vi "AO Reg UI.vi"(8 "error in (no error)":errorcluster, 11 "Node Ptr":T4 format="%.0x") -> (0 "error out":errorcluster)   [LabVIEW 2019, in "Modbus Master System Explorer.lvlib"]
uses:
  Modbus Master System Explorer.lvlib
  <vilib>/NI VeriStand/Custom Device API/Custom Device Item Ref.ctl
  Shared/Controls/Data Model/DataType.ctl
  SubVIs/Radix.ctl
  SubVIs/Direction.ctl
  <vilib>/NI VeriStand/Custom Device API/Custom Device API.lvlib
  Shared/Modbus Master Shared.lvlib
panel:
  in  "Default Value":dbl
  in  "Direction":T1
  in  "Radix":T2
  out "Registers":i32
  in  "Sub-Index (Bool)":u16
  in  "DataType":T3
  in  "Valid?":string
  in  "Address":u16
  in  "Header":cluster{"Section Name":string}={"Section Name"="Holding Register (Analog Out) Settings"}
  in  "Description":string
  in  "Name":string
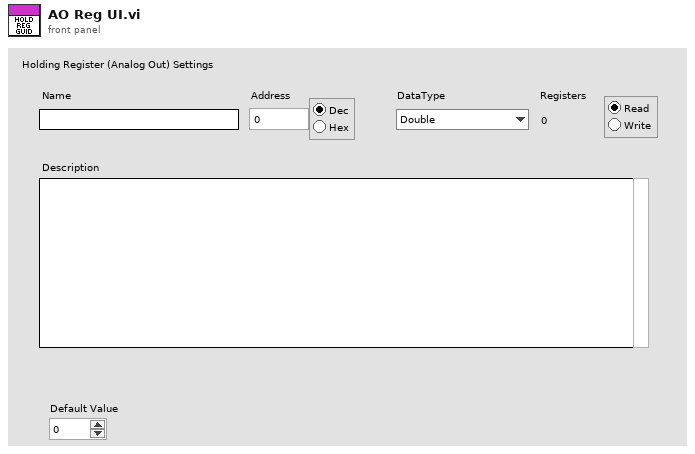
[diagram p1: front panel]
types:
  T1 = typedef "Modbus Master System Explorer.lvlib/Direction.ctl" = enum32{"Radio Selection 1", "Radio Selection 2"}
  T2 = typedef "Modbus Master System Explorer.lvlib/Radix.ctl" = enum32{"Decimal", "Hexidecimal"}
  T3 = typedef "Modbus Master Shared.lvlib/DataType.ctl" = enum16{"Double", "Single", "I64", "I32", "I16", "I8", "U64", "U32", "U16", "U8", "Boolean"}
  T4 = typedef "Custom Device API.lvlib/Custom Device Item Ref.ctl" = u64
  T5 = enum8{"Enabled", "Disabled", "Disabled and Grayed Out"}
  T6 = typedef "Custom Device API.lvlib/Custom Device Commands.ctl" = enum16{"Default", "Item renamed", "Shutdown", "Dynamic button pressed"}
  T7 = typedef "Custom Device API.lvlib/Custom Device Item Info.ctl" = cluster{"Name":string, "Is Channel":bool, "GUID":string, "Is Waveform":bool}
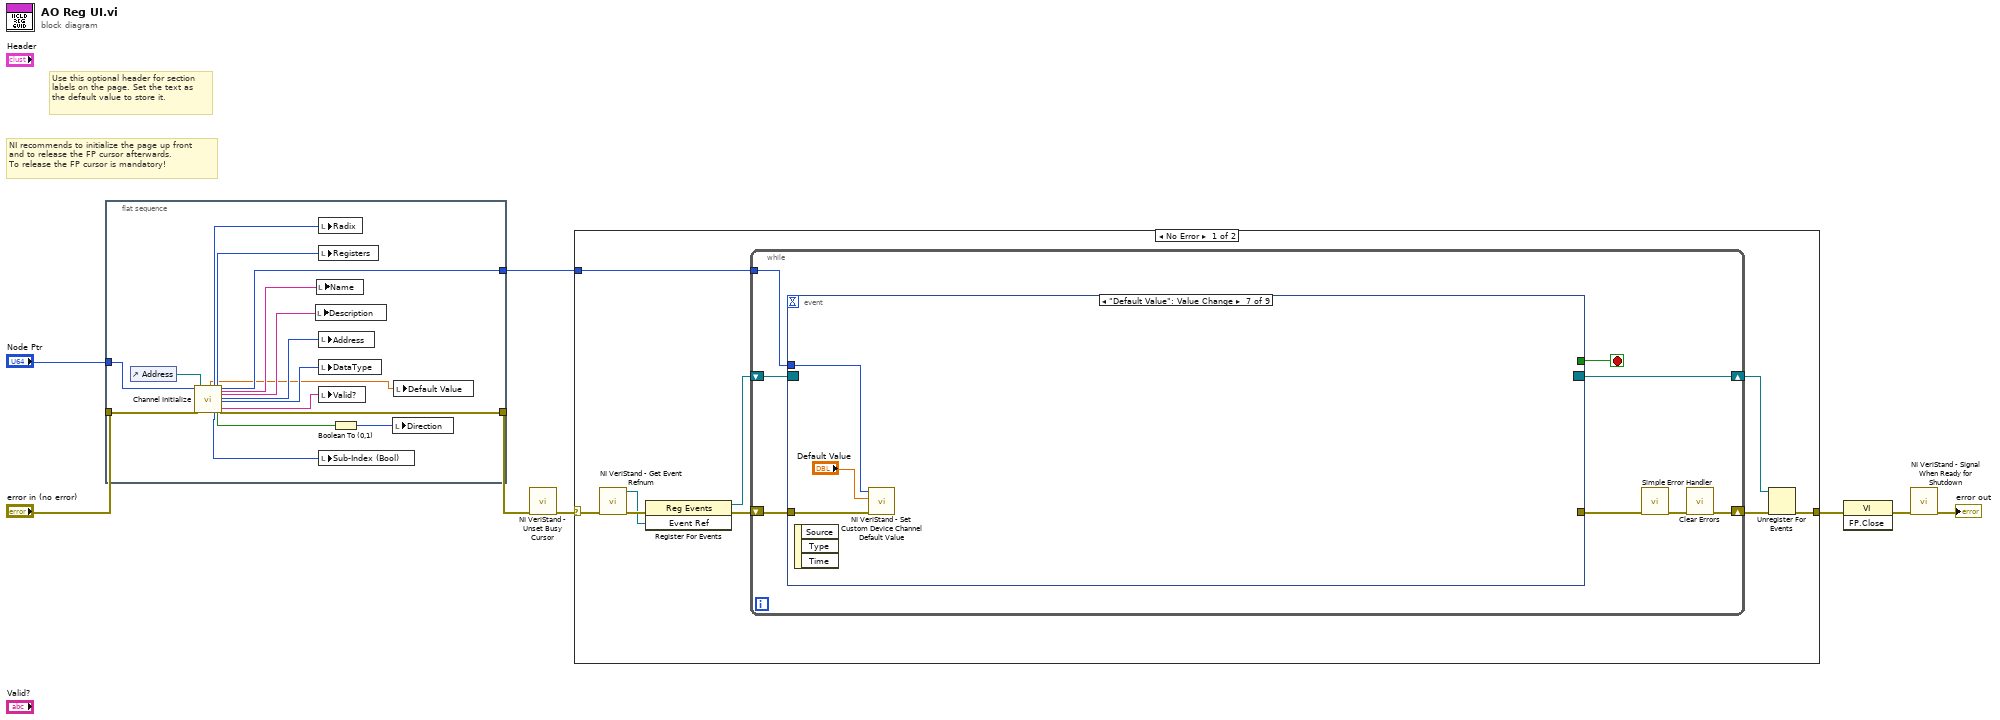
[diagram p0: block diagram]
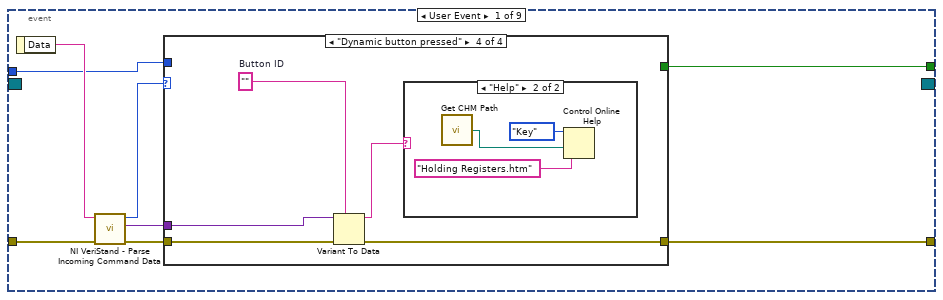
[diagram p2: hidden frame]
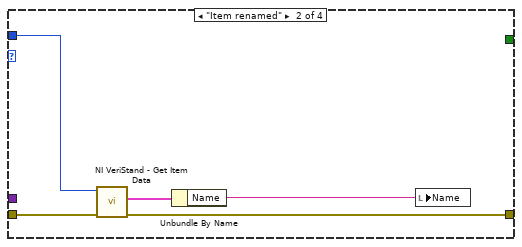
[diagram p4: hidden frame]
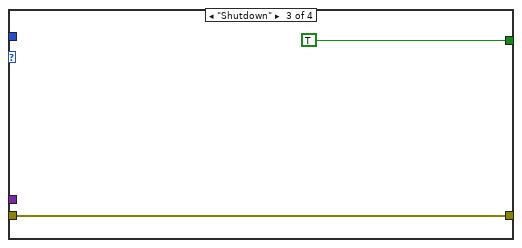
[diagram p5: hidden frame]
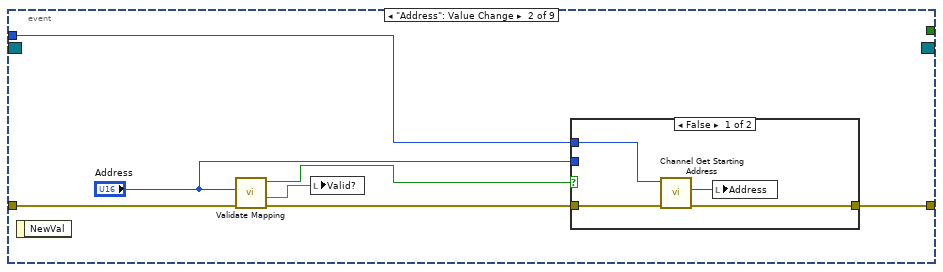
[diagram p7: hidden frame]
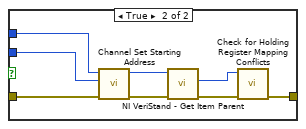
[diagram p8: hidden frame]
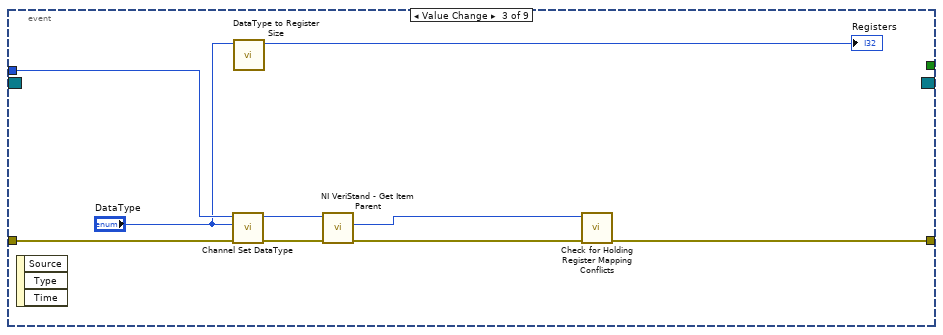
[diagram p9: hidden frame]
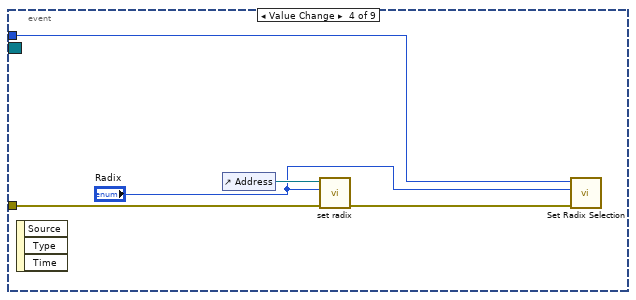
[diagram p10: hidden frame]
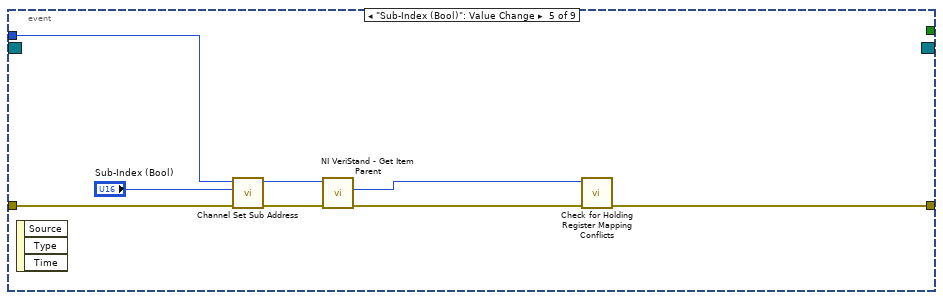
[diagram p11: hidden frame]
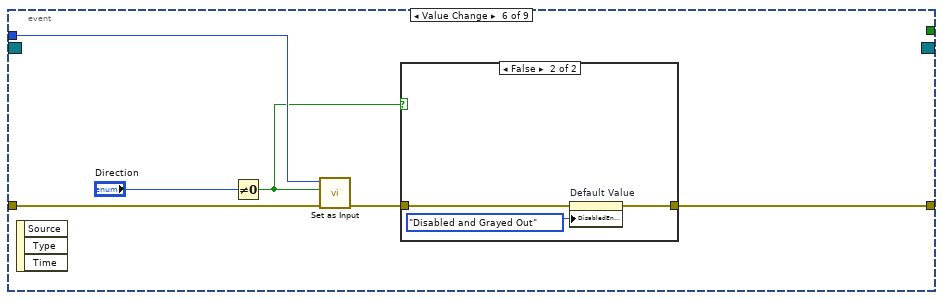
[diagram p12: hidden frame]
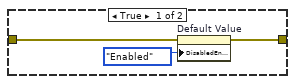
[diagram p13: hidden frame]
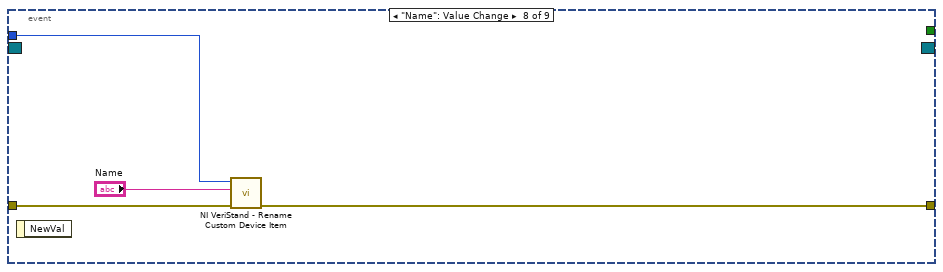
[diagram p14: hidden frame]
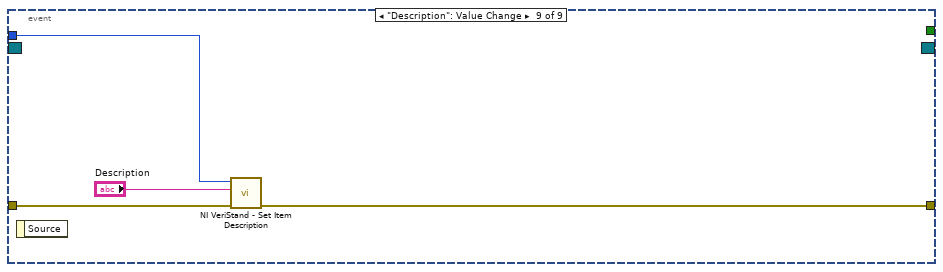
[diagram p15: hidden frame]
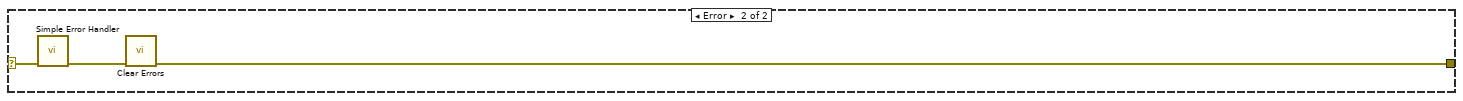
[diagram p16: hidden frame]
diagram:
  # "Use this optional header for section labels on the page. Set the text as the default value to store it."
  # "NI recommends to initialize the page up front\nand to release the FP cursor afterwards.\nTo release the FP cursor is mandatory!"
  n1 = flat-sequence {
    tunnel: "Node Ptr" -> [w13]
    tunnel: "error in (no error)" -> [w12]
    tunnel: [w11] -> w2
    tunnel: [w10] -> w1
    frame #0 {
      n2 = control-ref of="Address"() -> (w17:refnum<vi>)
      n3 = call "Channel Initialize.vi"("Item Ref in"=w13, "error in (no error)"=w12, "Starting Address Ref in"=w17) -> ("Default Value"=w9:dbl, "Radix"=w16:T2, "Sub-Index (Bool)"=w19:u16, "Registers"=w20:i32, "input?"=w14:bool, "Channel Ref out"=w11:T4, "Name"=w23:string, "Description"=w24:string, "Starting Address"=w21:u16, "DataType"=w22:T3, "Status Message"=w18:string, "error out"=w10:errorcluster)  [unwired: 12 in, 1 out]
      n4 = local write "Description"(w24) -> ()
      n5 = local write "Name"(w23) -> ()
      n6 = local write "Radix"(w16) -> ()
      n7 = local write "Registers"(w20) -> ()
      n8 = local write "Address"(w21) -> ()
      n9 = local write "DataType"(w22) -> ()
      n10 = local write "Valid?"(w18) -> ()
      n11 = local write "Sub-Index (Bool)"(w19) -> ()
      n12 = Boolean To (0,1)(Boolean=w14) -> (0, 1=w15:i16)
      n13 = local write "Direction"(w15) -> ()
      n14 = local write "Default Value"(w9) -> ()
    }
  }
  n15 = call <vilib>:"NI VeriStand - Unset Busy Cursor.vi"("error in (no error)"=w1) -> ("error out"=w5:errorcluster)  [unwired: 10 out]
  n16 = case shown="No Error" w5 {
    selector: w5 -> [w25 w132]
    tunnel: [w30 w130] -> w8
    tunnel: w2 -> [w26 _]
    frame No Error {
      n17 = call <vilib>:"NI VeriStand - Get Event Refnum.vi"("error in (no error)"=w25) -> ("error out"=w33:errorcluster, "Event Ref"=w29:refnum<user-event>)  [unwired: 9 out]
      n18 = register-events(error in=w33, w29) -> (reference out=w27:refnum<event-registration>, error out=w28:errorcluster)  [unwired: 1 in]
      n19 = while {
        tunnel: w26 -> [w37]
        shift-right: [w34] -> w31
        shift-left: w28 -> [w40]
        shift-right: [w41] -> w32
        shift-left: w27 -> [w39]
        stop <- w38 stop-if-true
        n20 = event shown="[6] \"Default Value\": Value Change" {
          selector: w39 -> [_ _ _ _ _ _ _ _ _]
          dyn-events: [_ _ _ _ _ _ _ _ _] -> w41
          timeout: _ -> [_ _ _ _ _ _ _ _ _]
          tunnel: w40 -> [w49 w72 w93 w98 w104 w111 w119 w125 w128]
          tunnel: [w45 _ _ _ _ _ _ _ _] -> w38
          tunnel: [w44 w69 w87 _ w100 w108 _ w124 w127] -> w36
          tunnel: w37 -> [w43 w71 w92 w94 w106 w112 w120 w123 w129]
          event User Event {
            n21 = event-data() -> ("Data"=w48:string)  [unwired: 1 out]
            n22 = call <vilib>:"NI VeriStand - Parse Incoming Command Data.vi"("error in (no error)"=w49, "Incoming data"=w48) -> ("error out"=w47:errorcluster, "Outgoing data"=w42:variant, "Action"=w46:T6)  [unwired: 7 out]
            n23 = case shown="\"Dynamic button pressed\"" w46 {
              tunnel: w47 -> [w50 w55 w56 w62]
              tunnel: [_ _ TRUE _] -> w45
              tunnel: [w50 w52 w56 w59] -> w44
              tunnel: w43 -> [_ w54 _ _]
              tunnel: w42 -> [_ _ _ w61]
              frame "Default", Default {
              }
              frame "Item renamed" {
                n24 = call <vilib>:"NI VeriStand - Get Item Data.vi"("error in (no error)"=w55, "Item Ref in"=w54) -> ("error out"=w52:errorcluster, "Item Info"=w53:T7)  [unwired: 8 out]
                n25 = Unbundle By Name(w53) -> ("Name"=w51:string)
                n26 = local write "Name"(w51) -> ()
              }
              frame "Shutdown" {
              }
              frame "Dynamic button pressed" {
                w60 = ""  # Button ID
                n27 = Variant To Data(error in=w62, type=w60, Variant=w61) -> (data=w58:string, error out=w59:errorcluster)
                n28 = case shown="\"Help\"" w58 {
                  frame Default {
                  }
                  frame "Help" {
                    n29 = call "Get CHM Path.vi"() -> ("appended path"=w65:path)
                    n30 = Control Online Help(2:w65, 3:"Holding Registers.htm" ("String to search for"), 4:enum16{"Contents", "Key", "Close"}."Key" ("Operation")) -> ()  [unwired: 1 in, 1 out]
                  }
                }
              }
            }
          }
          event "Address": Value Change {
            n31 = event-data() -> ()  [unwired: 2 out]
            n32 = call "Validate Mapping.vi"("error in (no error)"=w72, "Mapping"="Address") -> ("error out"=w70:errorcluster, "Status Message"=w66:string, "Valid?"=w68:bool)  [unwired: 7 in]
            n33 = local write "Valid?"(w66) -> ()
            n34 = case shown="False" w68 {
              tunnel: w71 -> [w76 w83]
              tunnel: w70 -> [w75 w84]
              tunnel: [w74 w77] -> w69
              tunnel: "Address" -> [_ w82]
              frame False {
                n35 = call "Channel Get Starting Address.vi"("error in (no error)"=w75, "Item Ref in"=w76) -> ("error out"=w74:errorcluster, "Value"=w73:u16)  [unwired: 7 in, 1 out]
                n36 = local write "Address"(w73) -> ()
              }
              frame True {
                n37 = call "Channel Set Starting Address.vi"("error in (no error)"=w84, "Value"=w82, "Item Ref in"=w83) -> ("error out"=w81:errorcluster, "Item Ref out"=w80:T4)  [unwired: 7 in]
                n38 = call <vilib>:"NI VeriStand - Get Item Parent.vi"("error in (no error)"=w81, "Item Ref in"=w80) -> ("error out"=w78:errorcluster, "Parent Ref"=w79:T4)  [unwired: 6 in, 2 out]
                n39 = call "Check for Holding Register Mapping Conflicts.vi"("error in (no error)"=w78, "Group Ref in"=w79) -> ("error out"=w77:errorcluster)  [unwired: 6 in, 3 out]
              }
            }
          }
          event Value Change {
            n40 = event-data() -> ()  [unwired: 4 out]
            n41 = call "Channel Set DataType.vi"("error in (no error)"=w93, "DataType"="DataType", "Item Ref in"=w92) -> ("error out"=w88:errorcluster, "Item Ref out"=w90:T4)  [unwired: 7 in]
            n42 = call "DataType to Register Size.vi"("DataType"="DataType") -> ("Registers"=→"Registers":i32)  [unwired: 9 in, 1 out]
            n43 = call <vilib>:"NI VeriStand - Get Item Parent.vi"("error in (no error)"=w88, "Item Ref in"=w90) -> ("error out"=w89:errorcluster, "Parent Ref"=w91:T4)  [unwired: 6 in, 2 out]
            n44 = call "Check for Holding Register Mapping Conflicts.vi"("error in (no error)"=w89, "Group Ref in"=w91) -> ("error out"=w87:errorcluster)  [unwired: 6 in, 3 out]
          }
          event Value Change {
            n45 = event-data() -> ()  [unwired: 4 out]
            n46 = control-ref of="Address"() -> (w97:refnum<vi>)
            n47 = call "set radix.vi"("error in (no error)"=w98, "Radix"="Radix", "Digital in"=w97) -> ("error out"=w96:errorcluster)  [unwired: 8 in]
            n48 = call "Set Radix Selection.vi"("error in (no error)"=w96, "Radix"="Radix", "Item Ref in"=w94) -> ()  [unwired: 7 in, 2 out]
          }
          event "Sub-Index (Bool)": Value Change {
            n49 = event-data() -> ()  [unwired: 4 out]
            n50 = call "Channel Set Sub Address.vi"("error in (no error)"=w104, "Value"="Sub-Index (Bool)", "Item Ref in"=w106) -> ("error out"=w102:errorcluster, "Item Ref out"=w99:T4)  [unwired: 7 in]
            n51 = call <vilib>:"NI VeriStand - Get Item Parent.vi"("error in (no error)"=w102, "Item Ref in"=w99) -> ("error out"=w101:errorcluster, "Parent Ref"=w103:T4)  [unwired: 6 in, 2 out]
            n52 = call "Check for Holding Register Mapping Conflicts.vi"("error in (no error)"=w101, "Group Ref in"=w103) -> ("error out"=w100:errorcluster)  [unwired: 6 in, 3 out]
          }
          event Value Change {
            n53 = event-data() -> ()  [unwired: 4 out]
            n54 = Not Equal To 0?(x="Direction") -> (x != 0?=w107:bool)
            n55 = call "Set as Input.vi"("error in (no error)"=w111, "Direction"=w107, "Channel Ref in"=w112) -> ("error out"=w109:errorcluster)  [unwired: 7 in, 1 out]
            n56 = case shown="False" w107 {
              tunnel: w109 -> [w114 w117]
              tunnel: [w113 w116] -> w108
              frame True {
                n57 = property on="Default Value" class="DigNum (strict)"(error in=w114, "DisabledEnum"=T5."Enabled" ("Disabled")) -> (error out=w113:errorcluster)  [unwired: 1 in, 1 out]
              }
              frame False {
                n58 = property on="Default Value" class="DigNum (strict)"(error in=w117, "DisabledEnum"=T5."Disabled and Grayed Out" ("Disabled")) -> (error out=w116:errorcluster)  [unwired: 1 in, 1 out]
              }
            }
          }
          event "Default Value": Value Change {
            n59 = event-data() -> ()  [unwired: 4 out]
            n60 = call <vilib>:"NI VeriStand - Set Custom Device Channel Default Value.vi"("error in (no error)"=w119, "Default Value"="Default Value", "Channel Ref in"=w120) -> ()  [unwired: 7 in, 2 out]
          }
          event "Name": Value Change {
            n61 = event-data() -> ()  [unwired: 2 out]
            n62 = call <vilib>:"NI VeriStand - Rename Custom Device Item.vi"("error in (no error)"=w125, "New Name"="Name", "Item Ref in"=w123) -> ("error out"=w124:errorcluster)  [unwired: 1 in, 7 out]
          }
          event "Description": Value Change {
            n63 = event-data() -> ()  [unwired: 2 out]
            n64 = call <vilib>:"NI VeriStand - Set Item Description.vi"("error in (no error)"=w128, "Description"="Description", "Item Ref in"=w129) -> ("error out"=w127:errorcluster)  [unwired: 8 out]
          }
        }
        n65 = call <vilib>:"Simple Error Handler.vi"("error in (no error)"=w36) -> ("error out"=w35:errorcluster)  [unwired: 1 in, 7 out]
        n66 = call <vilib>:"Clear Errors.vi"("error in (no error)"=w35) -> ("error out"=w34:errorcluster)  [unwired: 1 in, 5 out]
      }
      n67 = Unregister For Events(event registration refnum=w32, error in=w31) -> (error out=w30:errorcluster)
    }
    frame Error {
      n68 = call <vilib>:"Simple Error Handler.vi"("error in (no error)"=w132) -> ("error out"=w131:errorcluster)  [unwired: 1 in, 7 out]
      n69 = call <vilib>:"Clear Errors.vi"("error in (no error)"=w131) -> ("error out"=w130:errorcluster)  [unwired: 1 in, 5 out]
    }
  }
  n70 = invoke class="VI" method="FP.Close"(error in=w8) -> (error out=w7:errorcluster)  [unwired: 2 in, 2 out]
  n71 = call <vilib>:"NI VeriStand - Signal When Ready for Shutdown.vi"("error in (no error)"=w7) -> ("error out"=→"error out":errorcluster)  [unwired: 10 out]
